vi "Autonomous.vi"   [LabVIEW 2020]
doc: "This VI starts when autonomous period begins, and will automatically be terminated when it ends. You can carry out timed or sensor driven operations directly to I/O or to subsystems without needing to return to the caller."
uses:
  Drive/Implementation/Robot Velocities.ctl
  <vilib>/Rock Robotics/WPI/Utilities/WPI_GetSetVariantRefNum.vi
  <vilib>/Rock Robotics/Network Tables/NT Read String.vi
types:
  T1 = typedef "WPI_JoystickDevRef.ctl" = cluster{"Device":T2}
  T2 = typedef "WPI_JoystickDeviceEnum.ctl" = enum16{"USB 0", "USB 1", "USB 2", "USB 3", "USB 4", "USB 5"}
  T3 = typedef "Robot Velocities.ctl" = cluster{"vx":dbl, "vy":dbl, "w":dbl}
  T4 = typedef "CTRE_PigeonIMU_DeviceRef.ctl" = cluster{"DeviceStatus":errorcluster, "Device Number":u8, "Type":T5, "Device ID":u32, "Handle":u64, "UsageFrame":u32, "Library Path":path}
  T5 = typedef "CTRE_PigeonIMU_ConnectionType.ctl" = u32
  T6 = typedef "Trajectory Data.ctl" = cluster{"Segment Name":string, "Type":T7, "Traj Pos Points":cluster{"x":dbl, "y":dbl, "th":dbl}[], "Traj Vel Points":cluster{"V":dbl, "Omega":dbl, "V vector":cluster{"y":dbl, "x":dbl}}[], "Accel Index":i32, "Decel Index":i32}[]
  T7 = typedef "Segment Type.ctl" = enum16{"Accel Straight", "Const Straight", "Blend", "Circle", "Bezier"}
  T8 = cluster{"V":dbl, "Omega":dbl, "V vector":cluster{"y":dbl, "x":dbl}}[]
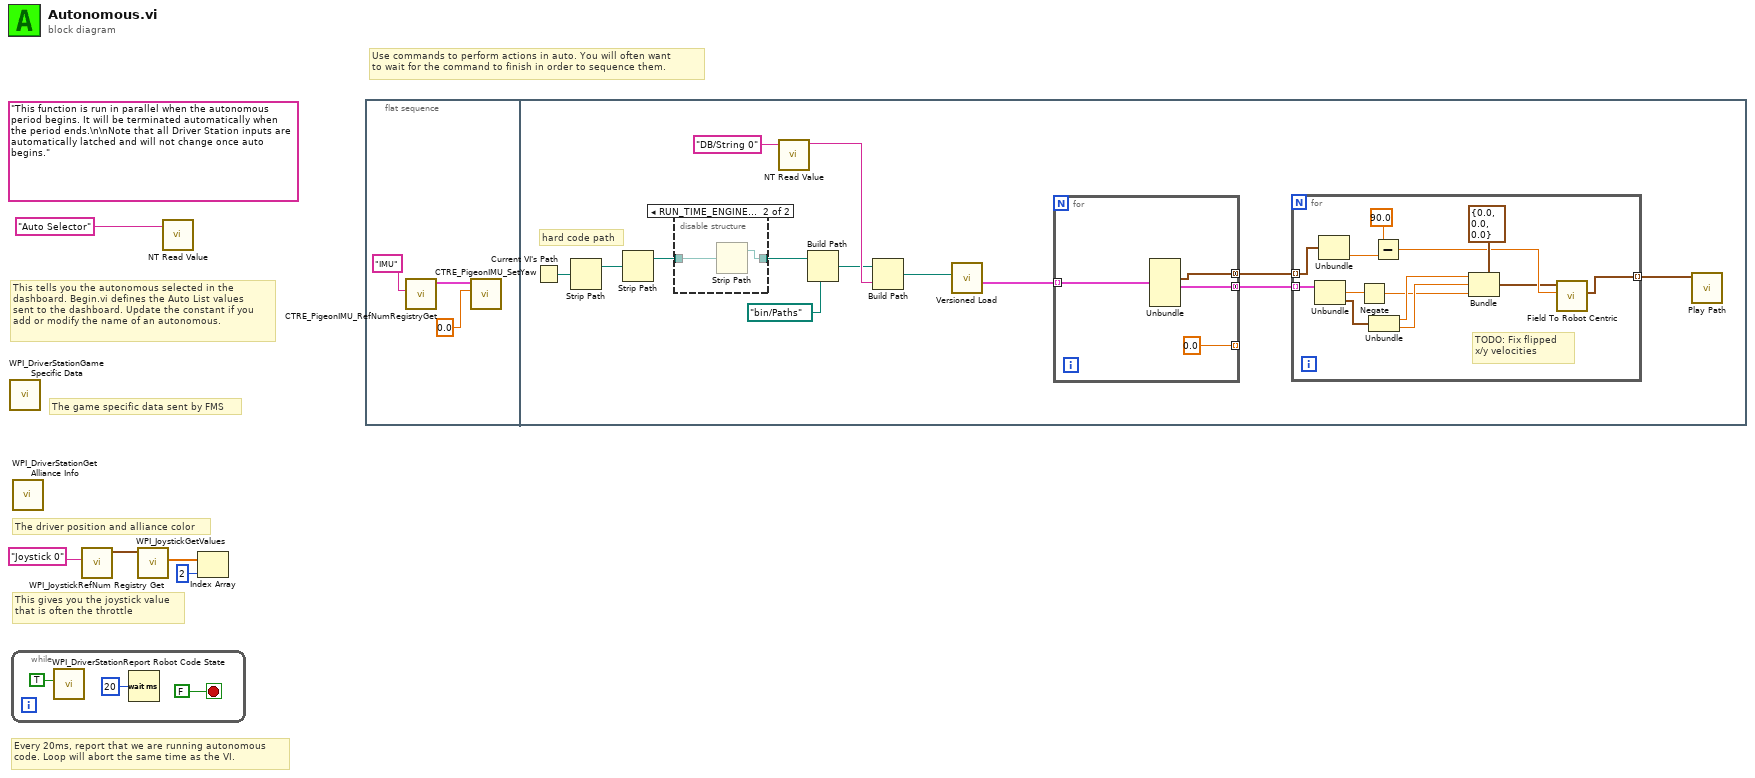
[diagram p0: block diagram]
diagram:
  (unwired) "This function is run in parallel when the autonomous period begins. It will be terminated automatically when the period ends.\n\nNote that all Driver Station inputs are automatically latched and will not change once auto begins."
  # "The game specific data sent by FMS"
  # "This tells you the autonomous selected in the \ndashboard. Begin.vi defines the Auto List values\nsent to the dashboard. Update the constant if you\nadd or modify the name of an autonomous."
  # "Every 20ms, report that we are running autonomous\ncode. Loop will abort the same time as the VI."
  # "This gives you the joystick value\nthat is often the throttle"
  # "Use commands to perform actions in auto. You will often want\nto wait for the command to finish in order to sequence them."
  # "The driver position and alliance color"
  n1 = call <vilib>:"WPI_DriverStationGame Specific Data.vi"() -> ()  [unwired: 11 in, 1 out]
  n2 = while {
    stop <- FALSE stop-if-true
    n3 = call <vilib>:"WPI_DriverStationReport Robot Code State.vi"("Autonomous"=TRUE) -> ()  [unwired: 10 in, 1 out]
    n4 = Wait (ms)(milliseconds to wait=u32 20) -> ()  [unwired: 1 out]
  }
  n5 = call <vilib>:"WPI_DriverStationGet Alliance Info.vi"() -> ()  [unwired: 12 out]
  n6 = call <vilib>:"WPI_JoystickRefNum Registry Get.vi"("refnum name"="Joystick 0") -> ("JoystickDevRef"=w4:T1)  [unwired: 1 in, 9 out]
  n7 = call <vilib>:"WPI_JoystickGetValues.vi"("JoystickDevRef"=w4) -> ("Axes"=w3:dbl[])  [unwired: 6 in, 4 out]
  n8 = call-poly <vilib>:"NT Read Value.vi"("name"="Auto Selector" ("Name")) -> ()  [unwired: 8 in, 3 out]
  n9 = Index Array(array=w3, index=2) -> ()  [unwired: 1 out]
  n10 = flat-sequence {
    frame #0 {
      n11 = call <vilib>:"CTRE_PigeonIMU_RefNumRegistryGet.vi"("refnum name"="IMU") -> ("PigeonIMUDevRef"=w11:T4)  [unwired: 9 in, 1 out]
      n12 = call <vilib>:"CTRE_PigeonIMU_SetYaw.vi"("Value"=0.0, "PigeonIMUDevRef"=w11) -> ()  [unwired: 8 in, 2 out]
    }
    frame #1 {
      # "hard code path"
      n13 = Current VI's Path() -> (path=w16:path)
      n14 = Strip Path(path=w16) -> (stripped path=w17:path)  [unwired: 1 out]
      n15 = Strip Path(path=w17) -> (stripped path=w19:path)  [unwired: 1 out]
      n16 = disable-structure shown="RUN_TIME_ENGINE==True, Default" {
        disable-tunnel: [w42 w43] -> w18
        disable-tunnel: w19 -> [w42 w44]
        frame condition #0 (active) {
        }
        frame condition #1 {
          n17 = Strip Path(path=w44) -> (stripped path=w43:path)  [unwired: 1 out]
        }
      }
      n18 = call-poly <vilib>:"NT Read Value.vi"("name"="DB/String 0" ("Name")) -> ("value"=w21:string)  [unwired: 8 in, 2 out]
      n19 = Build Path(base path=w18, name or relative path=path "bin/Paths") -> (appended path=w20:path)
      n20 = Build Path(base path=w20, name or relative path=w21) -> (appended path=w22:path)
      n21 = call "Versioned Load.vi"("path"=w22) -> ("Trajectory Data"=w23:T6)  [unwired: 3 in, 7 out]
      n22 = for {
        tunnel: w23 -> [w41] mode=indexing
        tunnel: [w40] -> w24 mode=concatenating
        tunnel: [0.0] -> _ mode=indexing
        tunnel: [w38] -> w13 mode=concatenating
        n23 = Unbundle(w41) -> ("Traj Pos Points"=w38:cluster{"x":dbl, "y":dbl, "th":dbl}[], "Traj Vel Points"=w40:T8)  [unwired: 4 out]
      }
      n24 = for {
        tunnel: w24 -> [w37] mode=indexing
        tunnel: w13 -> [w36] mode=indexing
        tunnel: [w27] -> w12 mode=indexing
        # "TODO: Fix flipped\nx/y velocities"
        n25 = Unbundle(w37) -> ("Omega"=w26:dbl, "V vector"=w35:cluster{"y":dbl, "x":dbl})  [unwired: 1 out]
        n26 = Unbundle(w36) -> ("th"=w31:dbl)  [unwired: 2 out]
        n27 = Negate(x=w26) -> (-x=w25:dbl)
        n28 = Unbundle(w35) -> ("y"=w33:dbl, "x"=w32:dbl)
        n29 = Subtract(x=90.0, y=w31) -> (x-y=w29:dbl)
        n30 = Bundle(cluster=T3 {"vx"=0.0, "vy"=0.0, "w"=0.0} ("Robot Velocities"), "vx"=w33, "vy"=w32, "w"=w25) -> (w28:T3)
        n31 = call "Field To Robot Centric.vi"("IMU Value (offset)"=w29, "Field Centric Velocities"=w28) -> ("Robot Centric Velocities"=w27:T3)  [unwired: 8 in, 1 out]
      }
      n32 = call "Play Path.vi"("Auto Velocities"=w12) -> ()  [unwired: 10 in, 1 out]
    }
  }
